vi "Read Bool A.vi"(8 "error in (no error)":errorcluster, 11 "Two Terminal in":refnum<class "AbsFunc_Two Term_Bool.lvclass">) -> (0 "error out":errorcluster, 2 "Abs_Types.lvlib:Boolean.lvclass":refnum<class "Abs_Boolean.lvclass">, 3 "Two Terminal out":refnum<class "AbsFunc_Two Term_Bool.lvclass">)   [LabVIEW 2021, in "AbsFunc_Two Term_Bool.lvclass"]
uses:
  AbsFunc_Two Term_Bool.lvclass
  Abs_Types/Boolean/Abs_Boolean.lvclass
  AbsFunc_Two Term_Bool.lvclass/AbsFunc_Two Term_Bool.ctl
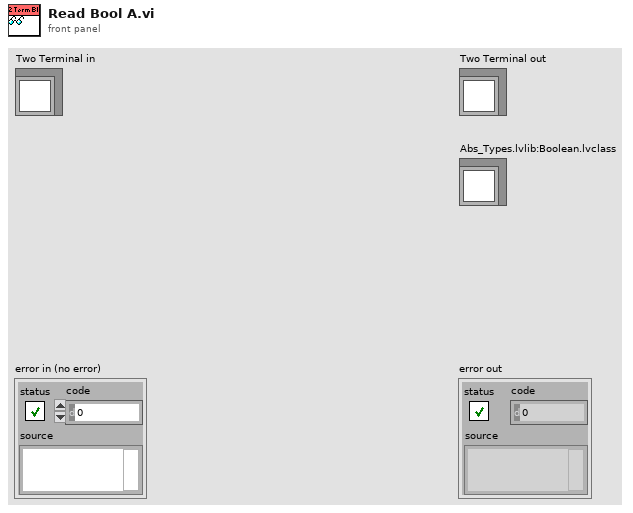
[diagram p1: front panel]
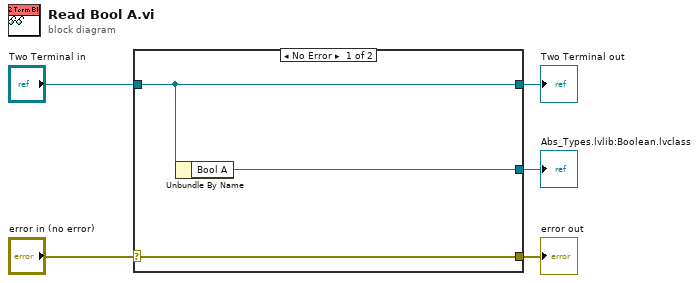
[diagram p0: block diagram]
diagram:
  n1 = case shown="No Error" "error in (no error)" {
    selector: "error in (no error)" -> [w8 w9]
    tunnel: [w8 w9] -> w4
    tunnel: [w7 w10] -> w2
    tunnel: "Two Terminal in" -> [w7 w10]
    tunnel: [w6 _] -> w1
    frame No Error {
      n2 = Unbundle By Name(w7) -> ("Bool A"=w6:refnum<class "Abs_Boolean.lvclass">)
    }
    frame Error {
    }
  }
  "error out" <- w4
  "Two Terminal out" <- w2
  "Abs_Types.lvlib:Boolean.lvclass" <- w1
